vi "Size Operations.vi"(8 "error in (no error)":errorcluster caption="entrée d'erreur (pas d'erreur)", 11 "Operations en entrée":refnum<class "Operations.lvclass"> caption="DNL_LabVIEW Object in") -> (0 "error out":errorcluster caption="sortie d'erreur", 1 "size":i32, 3 "Operations en sortie":refnum<class "Operations.lvclass"> caption="DNL_LabVIEW Object out")   [LabVIEW 2012, in "Operations.lvclass"]
uses:
  Operations.lvclass
  Operations.lvclass/Operations.ctl
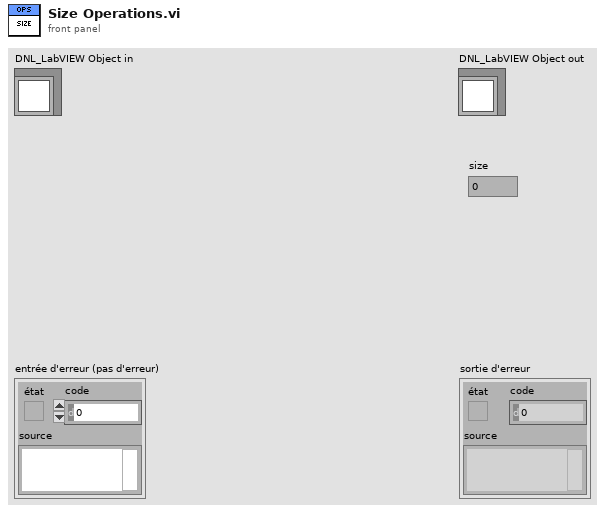
[diagram p1: front panel]
types:
  T1 = typedef "Dictionary Object RefNum__ogtk.ctl" = refnum<k1>
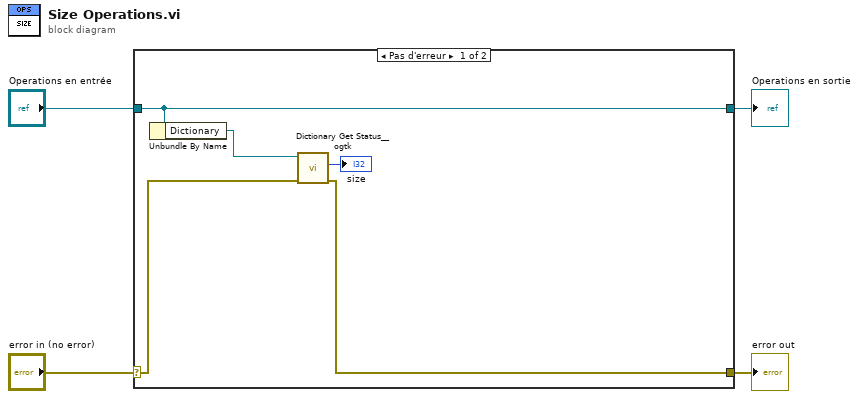
[diagram p0: block diagram]
diagram:
  n1 = case shown="Pas d'erreur" "error in (no error)" {
    selector: "error in (no error)" -> [w8 w11]
    tunnel: [w7 w11] -> w3
    tunnel: [w9 w10] -> w1
    tunnel: "Operations en entrée" -> [w9 w10]
    frame No Error {
      n2 = Unbundle By Name(w9) -> ("Dictionary"=w6:T1)
      n3 = call <userlib>:"Dictionary Get Status__ogtk.vi"("error in (no error)"=w8, "dictionary"=w6) -> ("error out"=w7:errorcluster, "size"=→"size":i32)  [unwired: 7 in, 1 out]
    }
    frame Error {
    }
  }
  "error out" <- w3
  "Operations en sortie" <- w1
